vi "CMD_08_Set_DAC_out.vi"(11 "DAC voltage, V":dbl min=-10.0 max=10.0) -> ()   [LabVIEW 2017]
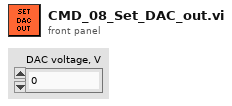
[diagram p1: front panel]
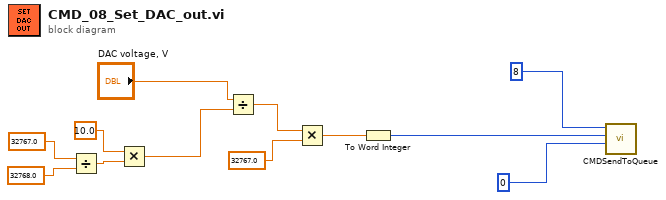
[diagram p0: block diagram]
diagram:
  n1 = Divide(x=32767.0, y=32768.0) -> (x/y=w3:dbl)
  n2 = Multiply(x=10.0 ("y"), y=w3) -> (x*y=w1:dbl)
  n3 = Divide(x="DAC voltage, V", y=w1) -> (x/y=w10:dbl)
  n4 = Multiply(x=w10, y=32767.0) -> (x*y=w11:dbl)
  n5 = To Word Integer(number=w11) -> (16bit integer=w7:i16)
  n6 = call "CMDSendToQueue.vi"("arg2"=i16 0, "arg1"=w7, "CMD"=i8 8) -> ()  [unwired: 9 in]
